vi "SWERVE_TRAJECTORY_EXECUTE.vi"(4 "Time Offset":dbl=-1.0 format="%16.4f", 6 "EnableClosedLoop":bool=TRUE, 7 "ABS_Traj ?":bool, 8 "Init":bool, 9 "Reverse":bool, 10 "Follow Orientation":bool, 11 "Gyro Heading\nRAD":dbl) -> (0 "AtReference":bool, 1 "OutputTRAJ_STATE":T6={"TimeSeconds"=0.0, "Velocity"=0.0, "Acceleration"=0.0, "POSE"={"TRANSLATION"={"X"=0.0, "Y"=0.0}, "ROTATION"={"VALUE"=0.0, "COS"=1.0, "SIN"=0.0}}, "Curvature"=0.0} {"POSE"."ROTATION"."SIN" format="%13.4f"; "POSE"."ROTATION"."COS" format="%13.4f"; "POSE"."ROTATION"."VALUE" format="%13.4f"; "POSE"."TRANSLATION"."Y" format="%14.3f"; "POSE"."TRANSLATION"."X" format="%14.3f"}, 2 "Error and Corr":T4 {"Error Pose"."ROTATION"."SIN" format="%13.4f"; "Error Pose"."ROTATION"."COS" format="%13.4f"; "Error Pose"."ROTATION"."VALUE" format="%13.4f"; "Error Pose"."TRANSLATION"."Y" format="%14.3f"; "Error Pose"."TRANSLATION"."X" format="%14.3f"}, 3 "Chassis Velocity Target":T5 {"vOmega" format="%10.3f"; "vY" format="%10.3f"; "vX" format="%10.3f"}, 5 "Orientation Target":dbl)   [LabVIEW 2023]
uses:
  <vilib>/Rock Robotics/WPI/ThirdParty/JAS_Junk/TrajLib/TypeDef/TRAJ_STATE.ctl
  <vilib>/Rock Robotics/WPI/ThirdParty/JAS_Junk/TrajLib/TypeDef/POSE2D.ctl
  <vilib>/Rock Robotics/WPI/ThirdParty/JAS_Junk/TrajLib/TypeDef/TRANSLATION2D.ctl
  <vilib>/Rock Robotics/WPI/ThirdParty/JAS_Junk/TrajLib/TypeDef/ROTATION2D.ctl
  <vilib>/Rock Robotics/WPI/ThirdParty/JAS_Junk/TrajLib/TypeDef/CHASSIS_SPEEDS.ctl
  <vilib>/Rock Robotics/WPI/ThirdParty/JAS_Junk/TrajLib/VI/Util_GetTime_U32.vi
  <vilib>/Rock Robotics/WPI/ThirdParty/JAS_Junk/TrajLib/MathUtil_InputModulus.vi
  <vilib>/Rock Robotics/WPI/ThirdParty/JAS_Junk/TrajLib/Rotation2d_UnaryMinus.vi
  <vilib>/Rock Robotics/WPI/ThirdParty/JAS_Junk/TrajLib/Rotation2d_RotateBy.vi
  <vilib>/Rock Robotics/WPI/ThirdParty/JAS_Junk/TrajLib/ProfiledPIDController_NewPeriod.vi
  <vilib>/Rock Robotics/WPI/ThirdParty/JAS_Junk/TrajLib/ProfiledPIDController_SetIntegratorRange.vi
  <vilib>/Rock Robotics/WPI/ThirdParty/JAS_Junk/TrajLib/ProfiledPIDController_DisableContInput.vi
  <vilib>/Rock Robotics/WPI/ThirdParty/JAS_Junk/TrajLib/ProfiledPIDController_EnableContInput.vi
  <vilib>/Rock Robotics/WPI/ThirdParty/JAS_Junk/TrajLib/TrapProfConstraint_New.vi
  <vilib>/Rock Robotics/WPI/ThirdParty/JAS_Junk/TrajLib/Rotation2d_Plus.vi
  <vilib>/Rock Robotics/WPI/ThirdParty/JAS_Junk/TrajLib/Twist2d_Create.vi
  <vilib>/Rock Robotics/WPI/ThirdParty/JAS_Junk/TrajLib/Pose2d_getTranslation.vi
  <vilib>/Rock Robotics/WPI/ThirdParty/JAS_Junk/TrajLib/VI/SwerveModulePosition_Get.vi
  <vilib>/Rock Robotics/WPI/ThirdParty/JAS_Junk/TrajLib/VI/SwerveModulePosition_New.vi
  <vilib>/Rock Robotics/WPI/ThirdParty/JAS_Junk/TrajLib/Twist2d_GetAll.vi
  <vilib>/Rock Robotics/WPI/ThirdParty/JAS_Junk/TrajLib/Translation2d_Create.vi
  <vilib>/Rock Robotics/WPI/ThirdParty/JAS_Junk/TrajLib/Conv_Deg_Radians.vi
  <vilib>/Rock Robotics/WPI/ThirdParty/JAS_Junk/TrajLib/HolDrvCtrl_New.vi
  <vilib>/Rock Robotics/WPI/ThirdParty/JAS_Junk/TrajLib/HolDrvCtrl_PackPID.vi
  <vilib>/Rock Robotics/WPI/ThirdParty/JAS_Junk/TrajLib/HolDrvCtrl_SetTolerance.vi
  <vilib>/Rock Robotics/WPI/ThirdParty/JAS_Junk/TrajLib/HolDrvCtrl_SetEnabled.vi
  <vilib>/Rock Robotics/WPI/ThirdParty/JAS_Junk/TrajLib/HolDrvCtrl_Calculate_Trajectory.vi
  <vilib>/Rock Robotics/WPI/ThirdParty/JAS_Junk/TrajLib/HolDrvCtrl_AtReference.vi
  <vilib>/Rock Robotics/WPI/ThirdParty/JAS_Junk/TrajLib/Translation2d_GetDistance.vi
  <vilib>/Rock Robotics/WPI/ThirdParty/JAS_Junk/TrajLib/Rotation2d_CreateXY.vi
  <vilib>/Rock Robotics/WPI/ThirdParty/JAS_Junk/TrajLib/TrapProfState_New.vi
  <vilib>/Rock Robotics/WPI/ThirdParty/JAS_Junk/TrajLib/PIDController_NewPeriod.vi
  <vilib>/Rock Robotics/SystemInterfaces/NetworkCommunication/NetComm_UsageReport_report.vi
  <vilib>/Rock Robotics/WPI/ThirdParty/JAS_Junk/TrajLib/PIDController_SetIntegratorRange.vi
  <vilib>/Rock Robotics/WPI/ThirdParty/JAS_Junk/TrajLib/PIDController_DisableContinousInput.vi
  <vilib>/Rock Robotics/WPI/ThirdParty/JAS_Junk/TrajLib/PIDController_EnableContinousInput.vi
  <vilib>/Rock Robotics/WPI/ThirdParty/JAS_Junk/TrajLib/PIDController_Reset.vi
  <vilib>/Rock Robotics/WPI/ThirdParty/JAS_Junk/TrajLib/HolDrvCtrl_Calculate.vi
  <vilib>/Rock Robotics/WPI/ThirdParty/JAS_Junk/TrajLib/Pose2d_getXYAngle.vi
  <vilib>/Rock Robotics/WPI/ThirdParty/JAS_Junk/TrajLib/Util_CalcDist.vi
  <vilib>/Rock Robotics/WPI/ThirdParty/JAS_Junk/TrajLib/Rotation2d_GetAngleCosSin.vi
  <vilib>/Rock Robotics/WPI/ThirdParty/JAS_Junk/TrajLib/Pose2d_RelativeTo.vi
  <vilib>/Rock Robotics/WPI/ThirdParty/JAS_Junk/TrajLib/ProfiledPIDController_Calculate_Meas_Goal.vi
  <vilib>/Rock Robotics/WPI/ThirdParty/JAS_Junk/TrajLib/PIDController_Calculate_SP_PV.vi
  <vilib>/Rock Robotics/WPI/ThirdParty/JAS_Junk/TrajLib/ProfiledPIDController_Reset_PosOnly.vi
  <vilib>/Rock Robotics/WPI/ThirdParty/JAS_Junk/TrajLib/ChassisSpeeds_FromFieldRelativeSpeeds.vi
  <vilib>/Rock Robotics/WPI/ThirdParty/JAS_Junk/TrajLib/Transform2d_Create_PosePose.vi
  <vilib>/Rock Robotics/WPI/ThirdParty/JAS_Junk/TrajLib/ProfiledPIDController_SetGoal_PosOnly.vi
  <vilib>/Rock Robotics/WPI/ThirdParty/JAS_Junk/TrajLib/ProfiledPIDController_Calculate_Meas.vi
  <vilib>/Rock Robotics/WPI/ThirdParty/JAS_Junk/TrajLib/PIDController_SetSetpoint.vi
  <vilib>/Rock Robotics/WPI/ThirdParty/JAS_Junk/TrajLib/PIDController_Calculate_PV.vi
  <vilib>/Rock Robotics/WPI/ThirdParty/JAS_Junk/TrajLib/ProfiledPIDController_Reset.vi
  <vilib>/Rock Robotics/WPI/ThirdParty/JAS_Junk/TrajLib/Rotation2d_GetCos.vi
  <vilib>/Rock Robotics/WPI/ThirdParty/JAS_Junk/TrajLib/Rotation2d_GetSin.vi
  <vilib>/Rock Robotics/WPI/ThirdParty/JAS_Junk/TrajLib/Translation2d_RotateBy.vi
  <vilib>/Rock Robotics/WPI/ThirdParty/JAS_Junk/TrajLib/Translation2d_Minus.vi
  <vilib>/Rock Robotics/WPI/ThirdParty/JAS_Junk/TrajLib/ProfiledPIDController_SetGoal.vi
  <vilib>/Rock Robotics/WPI/ThirdParty/JAS_Junk/TrajLib/TrapProfile_New.vi
  <vilib>/Rock Robotics/WPI/ThirdParty/JAS_Junk/TrajLib/ProfiledPIDController_GetPeriod.vi
  <vilib>/Rock Robotics/WPI/ThirdParty/JAS_Junk/TrajLib/TrapProfile_Calculate.vi
  <vilib>/Rock Robotics/WPI/ThirdParty/JAS_Junk/TrajLib/ControllerUtil_GetModulusError.vi
  <vilib>/Rock Robotics/WPI/ThirdParty/JAS_Junk/TrajLib/TrapProfile_ShouldFlipAcceleration.vi
  <vilib>/Rock Robotics/WPI/ThirdParty/JAS_Junk/TrajLib/TrapProfile_Direct.vi
  <vilib>/Rock Robotics/WPI/ThirdParty/JAS_Junk/TrajLib/PIDController_GetPeriod.vi
  <vilib>/Rock Robotics/WPI/ThirdParty/JAS_Junk/TrajLib/Globals/Util_LibraryGlobals.vi
  <vilib>/Rock Robotics/WPI/ThirdParty/JAS_Junk/TrajLib/VI/SwerveKinematics_ToTwist2dX.vi
  <vilib>/Rock Robotics/WPI/ThirdParty/JAS_Junk/TrajLib/Pose2d_Exp.vi
  <vilib>/Rock Robotics/SystemInterfaces/Utilities/FPGA_UtilitiesRead LocalTime.vi
  <vilib>/Rock Robotics/WPI/ThirdParty/JAS_Junk/TrajLib/VI/Util_GetTime_U64.vi
  <vilib>/Rock Robotics/WPI/ThirdParty/JAS_Junk/TrajLib/Trajectory_Library.lvlib
  <vilib>/Rock Robotics/WPI/ThirdParty/MJansen/PathPlanner/PathPlanner24.lvlib
panel:
  # "(FOR TESTING)"
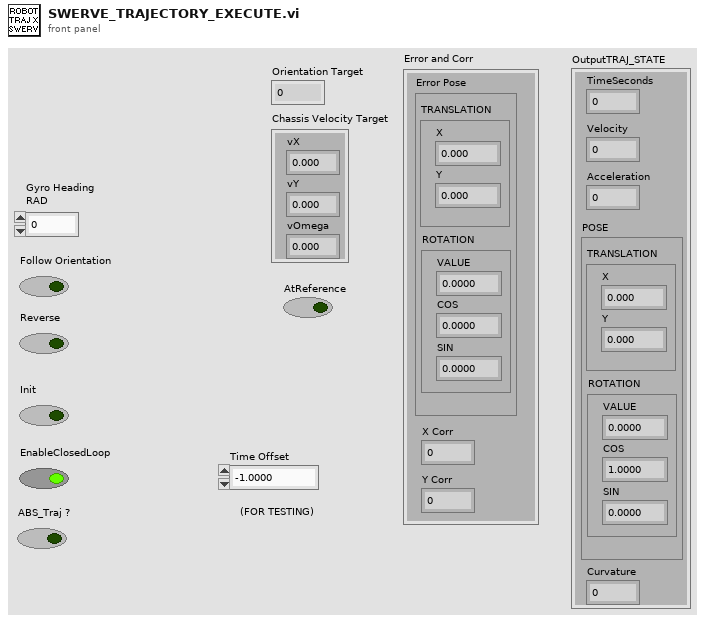
[diagram p1: front panel]
types:
  T1 = typedef "Trajectory_Library.lvlib/POSE2D.ctl" = cluster{"TRANSLATION":T2, "ROTATION":T3}
  T2 = typedef "Trajectory_Library.lvlib/TRANSLATION2D.ctl" = cluster{"X":dbl, "Y":dbl}
  T3 = typedef "Trajectory_Library.lvlib/ROTATION2D.ctl" = cluster{"VALUE":dbl, "COS":dbl, "SIN":dbl}
  T4 = cluster{"Error Pose":T1, "X Corr":dbl, "Y Corr":dbl}
  T5 = typedef "Trajectory_Library.lvlib/CHASSIS_SPEEDS.ctl" = cluster{"vX":dbl, "vY":dbl, "vOmega":dbl}
  T6 = typedef "Trajectory_Library.lvlib/TRAJ_STATE.ctl" = cluster{"TimeSeconds":dbl, "Velocity":dbl, "Acceleration":dbl, "POSE":T1, "Curvature":dbl}
  T7 = typedef "Trajectory_Library.lvlib/TRAJECTORY.ctl" = cluster{"TotalTImeSecs":dbl, "States":T6[]}
  T8 = typedef "PathPlanner24.lvlib/PathPlannerTrajectory.ctl" = cluster{"States":T9[]}
  T9 = typedef "PathPlanner24.lvlib/PathPlannerTrajectoryState.ctl" = cluster{"TimeSeconds":dbl, "VelocityMPS":dbl, "AccerationMpsSq":dbl, "HeadingAngularVelRadPerSec":dbl, "PositionMeters":T2, "Heading":T3, "TargetHolonomicRotation":T3, "CurvatureRadPerMeter":dbl, "PathPlannerConstraints":T10, "DeltaPos":dbl}
  T10 = typedef "PathPlanner24.lvlib/PathPlannerPathConstraints.ctl" = cluster{"MaxVelocityMps;":dbl, "MaxAccelerationMpsSq;":dbl, "MaxAngularVelRadPsEc;":dbl, "MaxAngularAccRadPSecSq":dbl, "Exists":bool}
  T11 = typedef "PathPlanner24.lvlib/PathPlannerPath.ctl" = cluster{"BezierPoints":T2[], "PreviewStartingRotation":T3, "Reversed":bool, "RotationTargets":T12[], "ConstraintZones":T13[], "EventMarkers":T14[], "GlobalConstraints":T10, "GoalEndState":T17, "AllPoints":T18[]}
  T12 = typedef "PathPlanner24.lvlib/PathPlannerRotationTarget.ctl" = cluster{"target":T3, "WaypointRelativePosition":dbl, "Exists":bool}
  T13 = typedef "PathPlanner24.lvlib/PathPlannerConstraintsZone.ctl" = cluster{"minWaypointPos":dbl, "maxWaypointPos":dbl, "Constraints":T10, "Present":bool}
  T14 = typedef "PathPlanner24.lvlib/PathPlannerEventMarker.ctl" = cluster{"WaypointRelativePos":dbl, "minimumTriggerDistance":dbl, "markerPos":T2, "lastRobotPos":T2, "Command":T15, "markerPos Exists":bool, "LastRobotPoseExists":bool, "Triggered":bool}
  T15 = typedef "PathPlanner24.lvlib/PathPlannerCommandUtil.ctl" = cluster{"waitTime":dbl, "name":string, "pathName":string, "commands":cluster{"type":T16, "waitTime":dbl, "name":string, "pathName":string}[], "type":T16}
  T16 = typedef "PathPlanner24.lvlib/PathPlanner_CommandUtilType_ENUM.ctl" = enum16{"Unknown", "Wait", "Named", "Path", "Sequential", "Parallel", "Race", "Deadline"}
  T17 = typedef "PathPlanner24.lvlib/PathPlannerGoalEndState.ctl" = cluster{"Velocity":dbl, "Rotation":T3}
  T18 = typedef "PathPlanner24.lvlib/PathPlannerPathPoint.ctl" = cluster{"Position":T2, "HolonomicRotation":T3, "DistAlongPath":dbl, "CurveRadius":dbl, "MaxV":dbl, "Constraints":T10, "HolonomicRotationExists":bool}
  T19 = typedef "Trajectory_Library.lvlib/SWERVE_DRIVE_KINEMATICS.ctl" = cluster{"NumModules":i32, "InverseKinematics":T20, "ForwardKinematics":T20, "Modules":T2[], "PrevCoR":T2, "SavedModuleStates":T21[]}
  T20 = typedef "NI_Matrix.lvlib/RealMatrix.ctl" = dbl[][]
  T21 = typedef "Trajectory_Library.lvlib/SWERVE_DRIVE_MODULE_STATE.ctl" = cluster{"Speed":dbl, "Angle":T3}
  T22 = typedef "Trajectory_Library.lvlib/SWERVE_DRIVE_ODOMETRY.ctl" = cluster{"POSE":T1, "GyroOffset":T3, "PreviousAngle":T3, "PrevModulePositions":T23[], "NumModules":i32}
  T23 = typedef "Trajectory_Library.lvlib/SWERVE_DRIVE_MODULE_POSITION.ctl" = cluster{"Distance":dbl, "Angle":T3, "P":bool}
  T24 = typedef "Trajectory_Library.lvlib/SWERVE_DRIVE_POSE_EST2.ctl" = cluster{"M_Vision_K":T20, "m_nominal_dT":dbl, "m_PrevTime_Sec":dbl, "Pose_Buffer":T25, "Swerve_Drive_Kinematics":T19, "Swerve_Drive_Odom":T22, "M_Q":T20, "NumModules":i32}
  T25 = typedef "Trajectory_Library.lvlib/TIME_INTERPOLATABLE_VARIANT.ctl" = cluster{"TimeStamps":dbl[], "DataArray":variant[], "Min_TimeStamp":dbl, "Max_TimeStamp":dbl, "ItemCount":i32, "MaxBufferTime":dbl}
  T26 = typedef "Trajectory_Library.lvlib/PID_TUNING.ctl" = cluster{"Kp":dbl, "Ki":dbl, "Kd":dbl, "MaximumIntegral":dbl, "MinimumIntegral":dbl, "IntegralZone":dbl}
  T27 = typedef "Trajectory_Library.lvlib/PROFILED_PID_CONTROLLER.ctl" = cluster{"Controller":T28, "Goal":T29, "Setpoint":T29, "Constraint":T30}
  T28 = typedef "Trajectory_Library.lvlib/PID_CONTROLLER.ctl" = cluster{"Kp":dbl, "Ki":dbl, "Kd":dbl, "Period":dbl, "Max_Integral":dbl, "Min_Integral":dbl, "Max_Input":dbl, "Min_Input":dbl, "Continuous":bool, "PositionError":dbl, "VelocityError":dbl, "PrevError":dbl, "Total_Integral":dbl, "PositionTolerance":dbl, "VelocityTolerance":dbl, "SetPoint":dbl, "Kf":dbl, "Prev_Deriv":dbl, "Prev_Deriv 2":dbl, "DerivativeFilter":bool, "Min_Output":dbl, "Max_Output":dbl, "Prev_F_P":dbl, "Prev_F_P_2":dbl, "AntiWindupActive":bool, "Measurement":dbl, "IntegralZone":dbl}
  T29 = typedef "Trajectory_Library.lvlib/TRAPEZOID_PROFILE_STATE.ctl" = cluster{"Position":dbl, "Velocity":dbl}
  T30 = typedef "Trajectory_Library.lvlib/TRAPEZOID_PROFILE_CONSTRAINT.ctl" = cluster{"MaxVelocity":dbl, "MaxAcceleration":dbl}
  T31 = typedef "PathPlanner24.lvlib/PathPlannerReplanningConfig.ctl" = cluster{"enableInitialReplanning":bool, "enableDynamicReplanning":bool, "dynamicReplanningTotalErrorThreshold":dbl, "dynamicReplanningErrorSpikeThreshold":dbl}
  T32 = typedef "Trajectory_Library.lvlib/HOLONOMIC_PACK_TUNING.ctl" = cluster{"X PID Tuning":T26, "Y PID Tuning":T26, "thetaProfiledPID_CTRL":T27}
  T33 = typedef "PathPlanner24.lvlib/PathPlannerCmdFollowHolConfig.ctl" = cluster{"HOLONOMIC_CTRL_PACK_TUNING":T32, "Max Wheel Speed M/S":dbl, "Tolerance SI":T1, "Drive Base Radius M":dbl, "ControlPastEnd_Sec":dbl, "ReplanningConfig":T31, "Period_Sec":dbl, "Trigger Events":bool}
  T34 = typedef "Trajectory_Library.lvlib/HOLONOMIC_DRV_CTRL.ctl" = cluster{"poseTolerance":T1, "poseError":T1, "Enabled":bool, "PID_xCtrl":T28, "PID_yCtrl":T28, "PROF_PID_thetaCtrl":T27, "RotationError":T3, "FirstRun":bool}
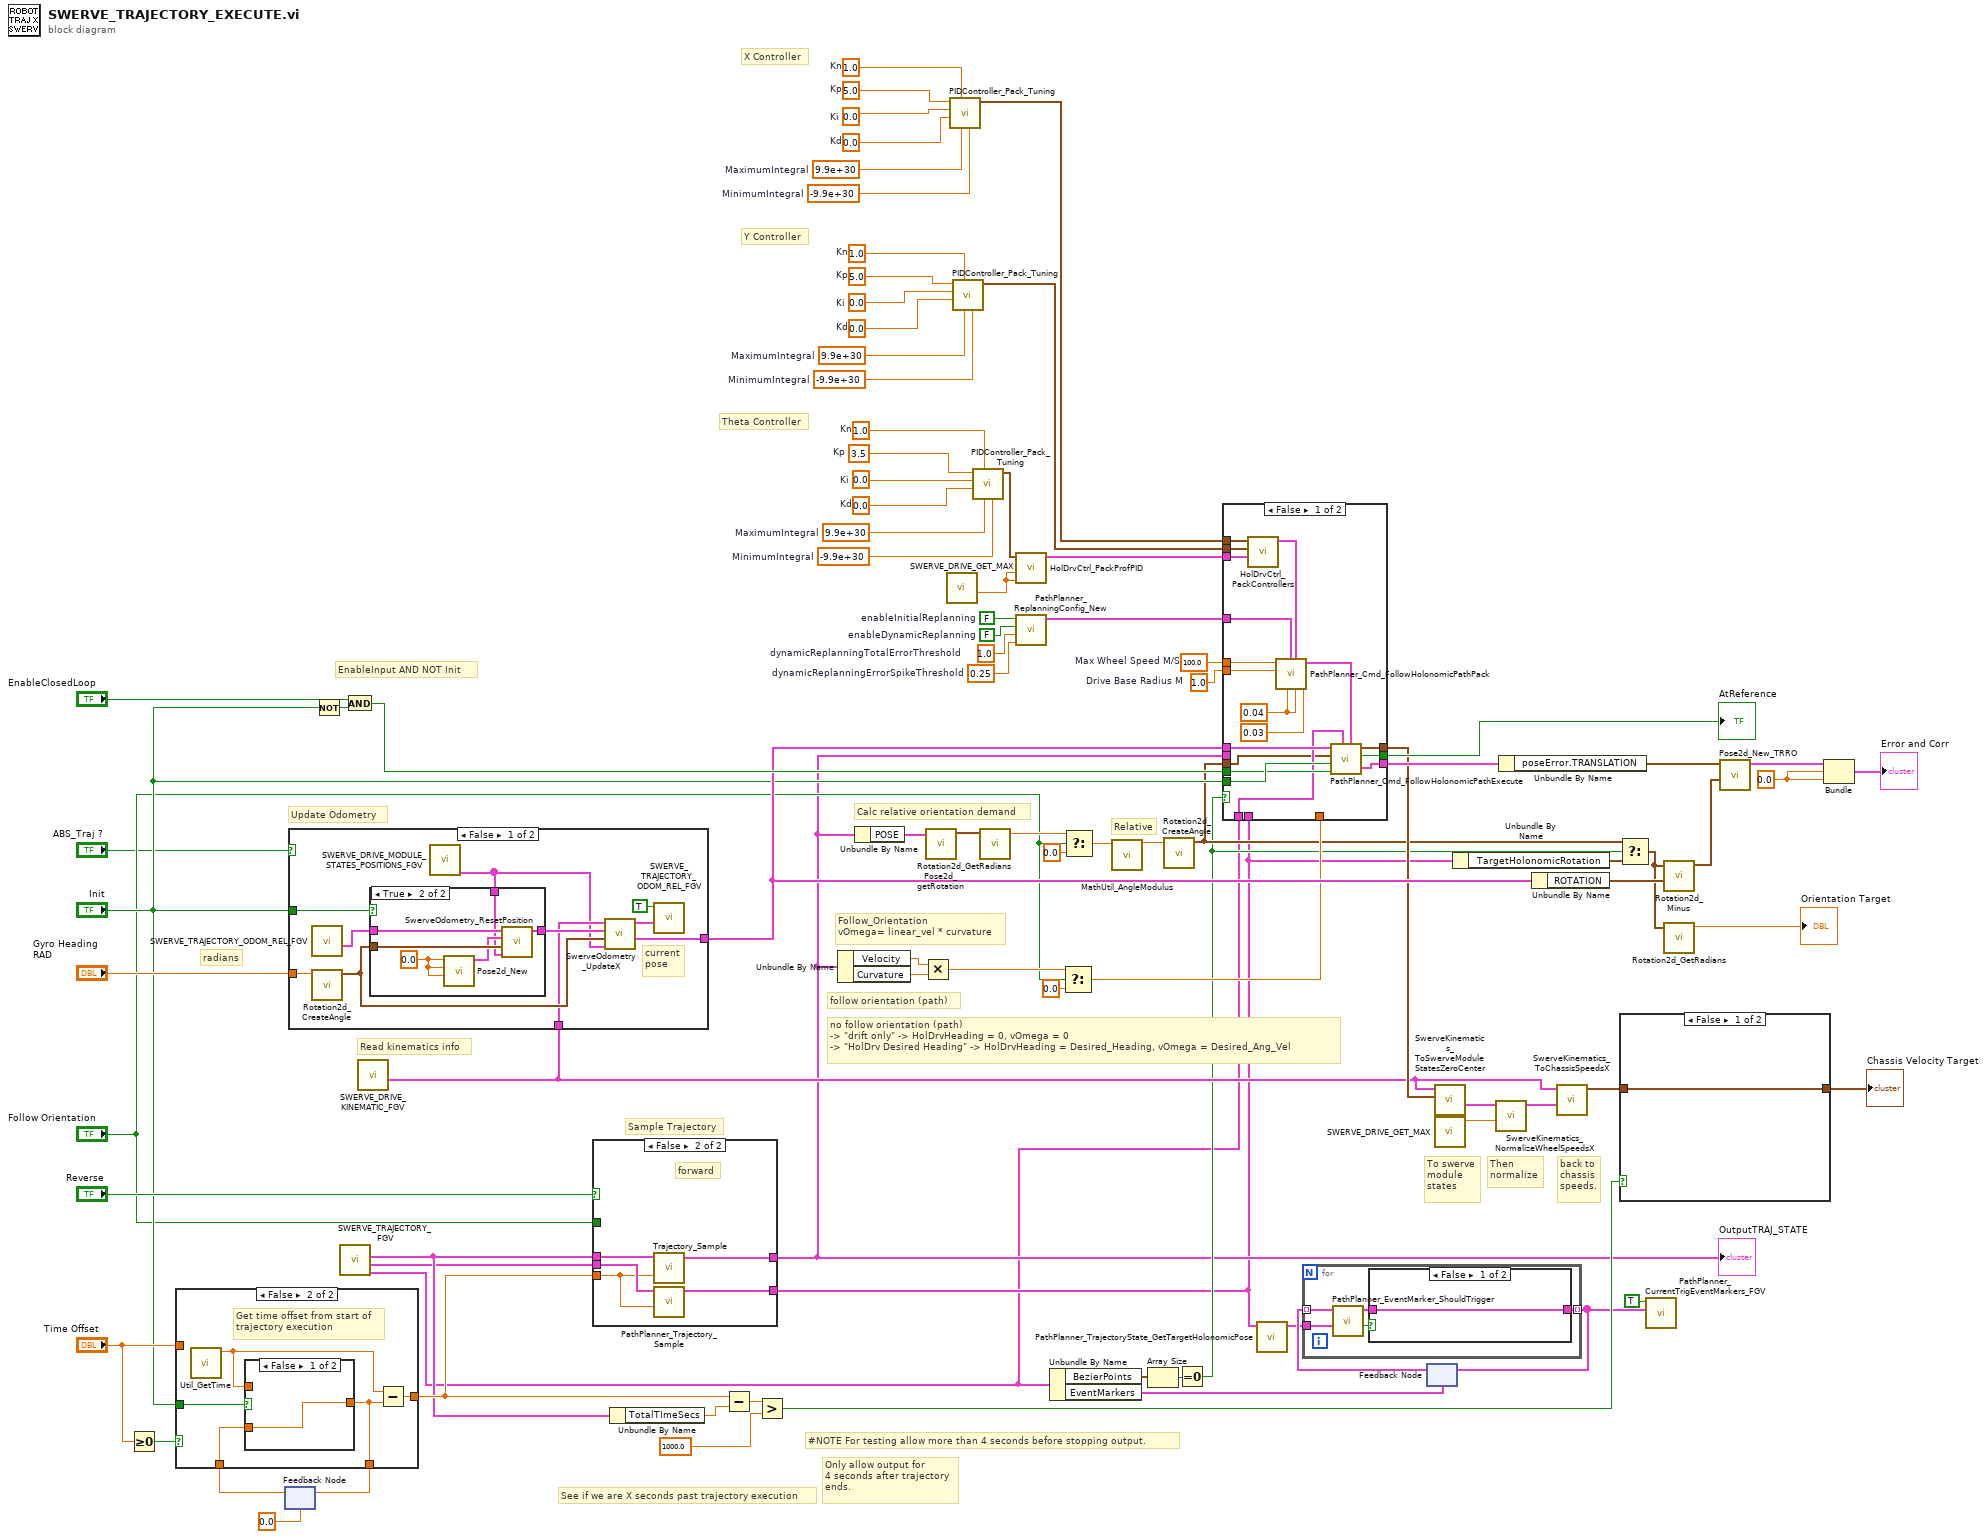
[diagram p0: block diagram]
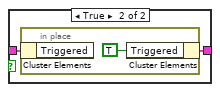
[diagram p2: hidden frame]
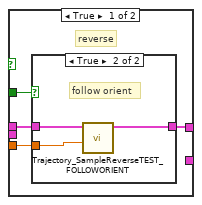
[diagram p3: hidden frame]
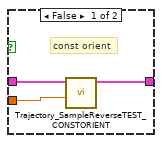
[diagram p4: hidden frame]
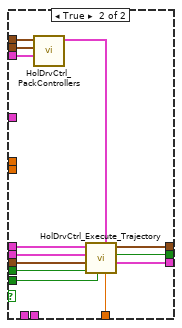
[diagram p5: hidden frame]
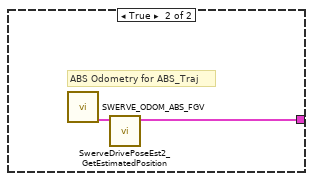
[diagram p7: hidden frame]
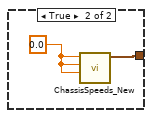
[diagram p10: hidden frame]
diagram:
  w7 = FALSE  # enableInitialReplanning
  w6 = FALSE  # enableDynamicReplanning
  w5 = 1.0  # dynamicReplanningTotalErrorThreshold
  w4 = 0.25  # dynamicReplanningErrorSpikeThreshold
  w21 = 1.0  # Drive Base Radius M
  w22 = 100.0  # Max Wheel Speed M/S
  w49 = 1.0  # Kn
  w52 = 3.5  # Kp
  w61 = 0.0  # Ki
  w62 = 0.0  # Kd
  w63 = 9.9e+30  # MaximumIntegral
  w64 = -9.9e+30  # MinimumIntegral
  w47 = 1.0  # Kn
  w50 = 5.0  # Kp
  w53 = 0.0  # Ki
  w54 = 0.0  # Kd
  w55 = 9.9e+30  # MaximumIntegral
  w56 = -9.9e+30  # MinimumIntegral
  w48 = 1.0  # Kn
  w51 = 5.0  # Kp
  w57 = 0.0  # Ki
  w58 = 0.0  # Kd
  w59 = 9.9e+30  # MaximumIntegral
  w60 = -9.9e+30  # MinimumIntegral
  w72 = 0.0
  # "Sample Trajectory"
  # "Update Odometry"
  # "Follow_Orientation\nvOmega= linear_vel * curvature"
  # "no follow orientation (path)\n-> \"drift only\" -> HolDrvHeading = 0, vOmega = 0\n-> \"HolDrv Desired Heading\" -> HolDrvHeading = Desired_Heading, vOmega = Desired_Ang_Vel"
  # "follow orientation (path)"
  # "#NOTE For testing allow more than 4 seconds before stopping output."
  # "EnableInput AND NOT Init"
  # "Theta Controller"
  # "Y Controller"
  # "X Controller"
  # "Relative"
  # "back to\nchassis\nspeeds."
  # "Then\nnormalize"
  # "To swerve\nmodule\nstates"
  # "Calc relative orientation demand"
  # "Read kinematics info"
  # "See if we are X seconds past trajectory execution"
  # "radians"
  # "Only allow output for\n4 seconds after trajectory\nends."
  n1 = Greater Or Equal To 0?(x="Time Offset") -> (x >= 0?=w76:bool)
  n2 = feedback #1(0.0 ("TIME")) -> (w78:dbl)
  n3 = case shown="False" w76 {
    tunnel: [w93 w99] -> w91
    tunnel: "Init" -> [_ w97]
    tunnel: w78 -> [w94 w96]
    tunnel: [w94 w95] -> w77
    tunnel: "Time Offset" -> [w93 _]
    frame True {
      # "For testing allow\nuser entered time offset!!"
    }
    frame False {
      # "Get time offset from start of\ntrajectory execution"
      n4 = call <vilib>:"Util_GetTime.vi"() -> ("FPGA_Time_Seconds"=w98:dbl)  [unwired: 9 in, 2 out]
      n5 = case shown="False" w97 {
        tunnel: [w100 w101] -> w95
        tunnel: w96 -> [w100 _]
        tunnel: w98 -> [_ w101]
        frame False {
        }
        frame True {
        }
      }
      n6 = Subtract(x=w98, y=w95) -> (x-y=w99:dbl)
    }
  }
  n7 = feedback-in #1(w77) -> ()
  n8 = Not(x="Init") -> (.not. x?=w73:bool)
  n9 = call "SWERVE_TRAJECTORY_FGV.vi"() -> ("outTRAJECTORY"=w24:T7, "outPathPlannerTrajectory"=w20:T8, "outPathPlannerPath"=w1:T11)  [unwired: 8 in]
  n10 = And(x="EnableClosedLoop", y=w73) -> (x .and. y?=w44:bool)
  n11 = call "SWERVE_DRIVE_KINEMATIC_FGV.vi"() -> ("out SWERVE_DRIVE_KINEMATICS"=w25:T19)  [unwired: 11 in]
  n12 = case shown="False" "ABS_Traj ?" {
    tunnel: "Gyro Heading\nRAD" -> [w111 _]
    tunnel: [w106 w119] -> w42
    tunnel: "Init" -> [w105 _]
    tunnel: w25 -> [w103 _]
    frame False {
      # "current\npose"
      n13 = call "SWERVE_TRAJECTORY_ODOM_REL_FGV.vi"() -> ("out SWERVE_DRIVE_ODOMETRY"=w110:T22)  [unwired: 11 in]
      n14 = call <vilib>:"Rotation2d_CreateAngle.vi"("Angle"=w111) -> ("ROTATION"=w104:T3)  [unwired: 10 in]
      n15 = call "SWERVE_DRIVE_MODULE_STATES_POSITIONS_FGV.vi"() -> ("out Current Module Positions"=w102:T23[])  [unwired: 10 in, 1 out]
      n16 = case shown="True" w105 {
        tunnel: w110 -> [w112 w118]
        tunnel: [w112 w117] -> w107
        tunnel: w104 -> [_ w116]
        tunnel: w102 -> [_ w113]
        frame False {
        }
        frame True {
          w115 = 0.0 ("X")
          n17 = call <vilib>:"Pose2d_New.vi"("Heading"=w115, "Y"=w115, "X"=w115) -> ("out POSe"=w114:T1)  [unwired: 8 in]
          n18 = call <vilib>:"SwerveOdometry_ResetPosition.vi"("Module Positions"=w113, "gyroAngle"=w116, "Pose"=w114, "in SWERVE_DRIVE_ODOMETRY"=w118) -> ("out SWERVE_DRIVE_ODOMETRY"=w117:T22)  [unwired: 6 in, 1 out]
        }
      }
      n19 = call <vilib>:"SwerveOdometry_UpdateX.vi"("module Positions"=w102, "gyroAngle"=w104, "in SWERVE_DRIVE_ODOMETRY"=w107, "SWERVE_DRIVE_KINEMATICS"=w103) -> ("robot POSE"=w106:T1, "out SWERVE_DRIVE_ODOMETRY"=w108:T22)  [unwired: 5 in, 1 out]
      n20 = call "SWERVE_TRAJECTORY_ODOM_REL_FGV.vi"("in SWERVE_DRIVE_ODOMETRY"=w108, "WRITE"=TRUE) -> ()  [unwired: 9 in, 1 out]
    }
    frame True {
      # "ABS Odometry for ABS_Traj"
      n21 = call "SWERVE_ODOM_ABS_FGV.vi"() -> ("out SWERVE_DRIVE_POSE_EST2"=w120:T24)  [unwired: 10 in, 1 out]
      n22 = call <vilib>:"SwerveDrivePoseEst2_GetEstimatedPosition.vi"("in SwerveDrivePoseEstimate"=w120) -> ("Estimated Pose"=w119:T1)  [unwired: 10 in]
    }
  }
  n23 = case shown="False" "Reverse" {
    tunnel: w24 -> [w124 w135]
    tunnel: w91 -> [w122 w132]
    tunnel: [w123 w134] -> w11
    tunnel: "Follow Orientation" -> [w121 _]
    tunnel: w20 -> [_ w133]
    tunnel: [_ w131] -> w9
    frame True {
      # "reverse"
      n24 = case shown="True" w121 {
        tunnel: w124 -> [w127 w130]
        tunnel: [w125 w129] -> w123
        tunnel: w122 -> [w126 w128]
        frame False {
          # "const orient"
          n25 = call "Trajectory_SampleReverseTEST_CONSTORIENT.vi"("Time"=w126, "InputTRAJECTORY"=w127) -> ("OutputTRAJ_STATE"=w125:T6)  [unwired: 9 in]
        }
        frame True {
          # "follow orient"
          n26 = call "Trajectory_SampleReverseTEST_FOLLOWORIENT.vi"("Time"=w128, "InputTRAJECTORY"=w130) -> ("OutputTRAJ_STATE"=w129:T6)  [unwired: 9 in]
        }
      }
    }
    frame False {
      # "forward"
      n27 = call <vilib>:"Trajectory_Sample.vi"("Time"=w132, "InputTRAJECTORY"=w135) -> ("OutputTRAJ_STATE"=w134:T6)  [unwired: 9 in]
      n28 = call <vilib>:"PathPlanner_Trajectory_Sample.vi"("Time"=w132, "PathPlannerTrajectory"=w133) -> ("PathPlannerState"=w131:T9)  [unwired: 9 in]
    }
  }
  "OutputTRAJ_STATE" <- w11
  n29 = Unbundle By Name(w24) -> ("TotalTImeSecs"=w92:dbl)
  n30 = Subtract(x=w91, y=w92) -> (x-y=w90:dbl)
  n31 = Greater?(x=w90, y=1000.0) -> (0:w88:bool)
  n32 = Unbundle By Name(w11) -> ("Velocity"=w32:dbl, "Curvature"=w31:dbl)
  n33 = Unbundle By Name(w11) -> ("POSE"=w80:T1)
  n34 = Multiply(x=w32, y=w31) -> (x*y=w29:dbl)
  n35 = call <vilib>:"Pose2d_getRotation.vi"("in POSE"=w80) -> ("out ROTATION"=w84:T3)  [unwired: 10 in]
  n36 = call "SWERVE_DRIVE_GET_MAX.vi"() -> ("Max Rotational Vel (Rad/Sec)"=w45:dbl)  [unwired: 10 in, 1 out]
  n37 = call <vilib>:"PIDController_Pack_Tuning.vi"("MinimumIntegral"=w56, "MaximumIntegral"=w55, "Kn"=w47, "Kd"=w54, "Ki"=w53, "Kp"=w50) -> ("PID Tuning"=w36:T26)  [unwired: 5 in]
  n38 = call <vilib>:"PIDController_Pack_Tuning.vi"("MinimumIntegral"=w60, "MaximumIntegral"=w59, "Kn"=w48, "Kd"=w58, "Ki"=w57, "Kp"=w51) -> ("PID Tuning"=w37:T26)  [unwired: 5 in]
  n39 = call <vilib>:"PIDController_Pack_Tuning.vi"("MinimumIntegral"=w64, "MaximumIntegral"=w63, "Kn"=w49, "Kd"=w62, "Ki"=w61, "Kp"=w52) -> ("PID Tuning"=w46:T26)  [unwired: 5 in]
  n40 = call <vilib>:"Rotation2d_GetRadians.vi"("in ROTATION"=w84) -> ("AngleRadians"=w43:dbl)  [unwired: 10 in]
  n41 = call <vilib>:"HolDrvCtrl_PackProfPID.vi"("Max Accel"=w45, "Max Speed"=w45, "Theta PID Tuning"=w46) -> ("Theta PID CONTROLLER"=w38:T27)  [unwired: 8 in]
  n42 = call <vilib>:"PathPlanner_ReplanningConfig_New.vi"("dynamicReplanningErrorSpikeThreshold"=w4, "dynamicReplanningTotalErrorThreshold"=w5, "enableDynamicReplanning"=w6, "enableInitialReplanning"=w7) -> ("ReplanningConfig"=w3:T31)  [unwired: 7 in]
  n43 = Unbundle By Name(w1) -> ("BezierPoints"=w19:T2[], "EventMarkers"=w12:T14[])
  n44 = Select(t=w29, s="Follow Orientation", f=0.0) -> (s? t:f=w27:dbl)
  n45 = Select(t=w43, s="Follow Orientation", f=0.0) -> (s? t:f=w65:dbl)
  n46 = call <vilib>:"MathUtil_AngleModulus.vi"("InputAngle"=w65) -> ("ModulsAngle"=w71:dbl)  [unwired: 10 in]
  n47 = Array Size(array=w19) -> (size(s)=w23:i32)
  n48 = call <vilib>:"Rotation2d_CreateAngle.vi"("Angle"=w71) -> ("ROTATION"=w17:T3)  [unwired: 10 in]
  n49 = Equal To 0?(x=w23) -> (x = 0?=w16:bool)
  n50 = case shown="False" w16 {
    tunnel: w44 -> [w144 w166]
    tunnel: w17 -> [w140 w165]
    tunnel: w42 -> [w146 w164]
    tunnel: [w142 w163] -> w41
    tunnel: [w147 w162] -> w40
    tunnel: [w143 w161] -> w39
    tunnel: w38 -> [w149 w160]
    tunnel: w37 -> [w150 w159]
    tunnel: w36 -> [w151 w158]
    tunnel: "Init" -> [w145 w156]
    tunnel: w11 -> [_ w155]
    tunnel: w27 -> [_ w154]
    tunnel: w22 -> [w153 _]
    tunnel: w21 -> [w152 _]
    tunnel: w9 -> [_ _]
    tunnel: w3 -> [w148 _]
    tunnel: w1 -> [w141 _]
    frame False {
      w138 = 0.04 ("X Tolerance M")
      n51 = call <vilib>:"HolDrvCtrl_PackControllers.vi"("thetaProfiledPID_CTRL"=w149, "Y PID Tuning"=w150, "X PID Tuning"=w151) -> ("HOLONOMIC_CTRL_PACK_TUNING"=w137:T32)  [unwired: 8 in]
      n52 = call <vilib>:"PathPlanner_Cmd_FollowHolonomicPathPack.vi"("Rotation Tolerance DEG"=0.03, "Y Tolerance M"=w138, "HOLONOMIC_CTRL_PACK_TUNING"=w137, "X Tolerance M"=w138, "ReplanningConfig"=w148, "Drive Base Radius M"=w152, "Max Wheel Speed M/S"=w153) -> ("PathPlanner_Ctrl_HolDrvConfig"=w136:T33)  [unwired: 4 in]
      n53 = call <vilib>:"PathPlanner_Cmd_FollowHolonomicPathExecute.vi"("PathPlanner_Cmd_FollowHolConfig"=w136, "PathPlannerPath"=w141, "Enabled"=w144, "Reset"=w145, "CurrentChassisSpeeds"=w140, "Current Pose SI"=w146) -> ("At Reference"=w142:bool, "calcChassisSpeed"=w143:T5, "outHOLONOMIC_DRV_CTRL"=w147:T34)  [unwired: 1 in, 2 out]
    }
    frame True {
      n54 = call <vilib>:"HolDrvCtrl_PackControllers.vi"("thetaProfiledPID_CTRL"=w160, "Y PID Tuning"=w159, "X PID Tuning"=w158) -> ("HOLONOMIC_CTRL_PACK_TUNING"=w157:T32)  [unwired: 8 in]
      n55 = call <vilib>:"HolDrvCtrl_Execute_Trajectory.vi"("Rotational Velocity Feedforward \nRad/Sec"=w154, "HOLONOMIC_CTRL_PACK_TUNING"=w157, "Reset"=w156, "Enable"=w166, "angleRef"=w165, "desiredTrajState"=w155, "currentPose"=w164) -> ("outHOLONOMIC_DRV_CTRL"=w162:T34, "AtReference"=w163:bool, "calcChassisSpeed"=w161:T5)  [unwired: 2 in]
    }
  }
  "AtReference" <- w41
  n56 = call <vilib>:"PathPlanner_TrajectoryState_GetTargetHolonomicPose.vi"("PathPlannerState"=w9) -> ("TargetHolonomicPose"=w8:T1)  [unwired: 10 in]
  n57 = feedback #2(w12) -> (w13:T14[])
  n58 = for {
    tunnel: w13 -> [w171] mode=indexing
    tunnel: w8 -> [w170]
    tunnel: [w167] -> w2 mode=indexing
    n59 = call <vilib>:"PathPlanner_EventMarker_ShouldTrigger.vi"("RobotPose"=w170, "in EventMarker"=w171) -> ("ShouldTrigger"=w168:bool, "out EventMarker"=w169:T14)  [unwired: 8 in]
    n60 = case shown="False" w168 {
      tunnel: w169 -> [w172 w174]
      tunnel: [w172 w173] -> w167
      frame False {
      }
      frame True {
        n61 = in-place {
          n62 = in-place-cluster #3(w174) -> ()  [unwired: 1 out]
          n63 = in-place-cluster #3("Triggered"=TRUE) -> (w173:T14)
        }
      }
    }
  }
  n64 = feedback-in #2(w2) -> ()
  n65 = call <vilib>:"SwerveKinematics_ToSwerveModuleStatesZeroCenter.vi"("ChassisSpeeds"=w39, "in SWERVE_DRIVE_KINEMATICS"=w25) -> ("ModuleStates"=w86:T21[])  [unwired: 8 in, 1 out]
  n66 = call "SWERVE_DRIVE_GET_MAX.vi"() -> ("Max Wheel Vel (Meter/Sec)"=w81:dbl)  [unwired: 10 in, 1 out]
  n67 = Unbundle By Name(w9) -> ("TargetHolonomicRotation"=w18:T3)
  n68 = call <vilib>:"SwerveKinematics_NormalizeWheelSpeedsX.vi"("AttainableMaxSpeed"=w81, "in WheelStates"=w86) -> ("out WheelStates"=w85:T21[])  [unwired: 9 in]
  n69 = Unbundle By Name(w40) -> ("poseError.TRANSLATION"=w70:T2)
  n70 = Unbundle By Name(w42) -> ("ROTATION"=w66:T3)
  n71 = call <vilib>:"SwerveKinematics_ToChassisSpeedsX.vi"("WheelStates"=w85, "in SWERVE_DRIVE_KINEMATICS"=w25) -> ("Chassis Speed"=w33:T5)  [unwired: 9 in]
  n72 = Select(t=w17, s=w16, f=w18) -> (s? t:f=w15:T3)
  n73 = case shown="False" w88 {
    tunnel: w33 -> [w176 _]
    tunnel: [w176 w177] -> w82
    frame False {
    }
    frame True {
      w178 = 0.0 ("vX")
      n74 = call <vilib>:"ChassisSpeeds_New.vi"("vAngular"=w178, "vY"=w178, "vX"=w178) -> ("CHASSIS"=w177:T5)  [unwired: 8 in]
    }
  }
  "Chassis Velocity Target" <- w82
  n75 = call "PathPlanner_CurrentTrigEventMarkers_FGV.vi"("in EventMarkers"=w2, "Write"=TRUE) -> ()  [unwired: 9 in, 1 out]
  n76 = call <vilib>:"Rotation2d_Minus.vi"("other ROTATION"=w66, "in ROTATION"=w15) -> ("out ROTATION"=w69:T3)  [unwired: 9 in]
  n77 = call <vilib>:"Rotation2d_GetRadians.vi"("in ROTATION"=w15) -> ("AngleRadians"=→"Orientation Target":dbl)  [unwired: 10 in]
  n78 = call <vilib>:"Pose2d_New_TRRO.vi"("ROTATION"=w69, "TRANSLATION"=w70) -> ("outPOSE"=w68:T1)  [unwired: 9 in]
  n79 = Bundle("outPOSE"=w68, w72, w72) -> (→"Error and Corr":cluster{"outPOSE":T1, dbl, dbl})  [unwired: 1 in]
